vi "QDMH POLY Enqueue Clusters.vi"(8 "error in (no error)":errorcluster, 10 "QDSM Elements":T1(array[cluster]), 11 "queue":refnum<queue>) -> (0 "error out":errorcluster, 3 "queue out":refnum<queue>)   [LabVIEW 2019]
doc: "This is an instance VI for the polymorphic enqueue VI.\n\nAAL 9/09"
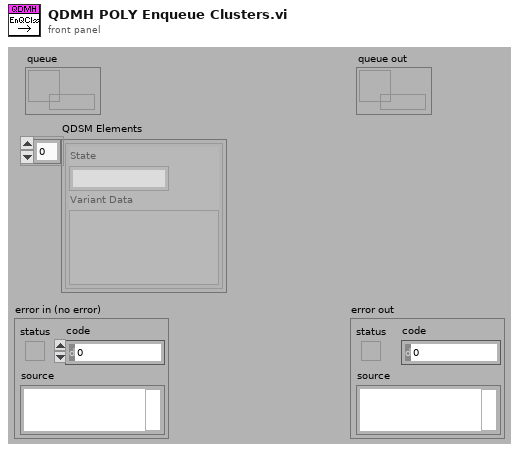
[diagram p1: front panel]
types:
  T1 = cluster{"State":string, "Variant Data":variant}[]
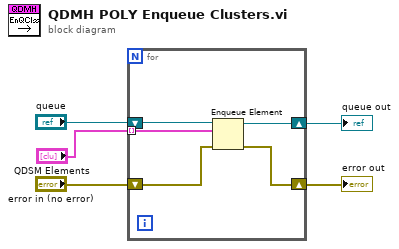
[diagram p0: block diagram]
diagram:
  n1 = for {
    tunnel: "QDSM Elements" -> [w6] mode=indexing
    shift-right: [w9] -> w4
    shift-left: "queue" -> [w10]
    shift-right: [w7] -> w2
    shift-left: "error in (no error)" -> [w8]
    n2 = Enqueue Element(queue=w10, element=w6, error in (no error)=w8) -> (queue out=w9:refnum<queue>, error out=w7:errorcluster)  [unwired: 2 out]
  }
  "queue out" <- w4
  "error out" <- w2
